vi "Configure Acquisition.vi"(7 "Continuous Storage (T: Enable)":bool=TRUE, 8 "error in (no error)":errorcluster, 10 "Sample Rate (0: 62.5 mHz)":u16(ring) items=["62.5 mHz", "125 mHz", "250 mHz", "500 mHz", "1 Hz", "2 Hz", "4 Hz", "8Hz", "16 Hz", "32 Hz", "64 Hz", "128 Hz", "256 Hz", "512 Hz", "Trigger "], 11 "VISA resource name":refnum<visa-resource-name>) -> (0 "error out":errorcluster, 3 "VISA resource name out":refnum<visa-resource-name>)   [LabVIEW 2020, in "Stanford Research 830.lvlib"]
doc: "Configures the storage of the acquired data in the internal buffer.\n\n<B>Note:</B>\n\nThis VI configures how the data is acquired and stored from the display to the internal buffer of the instrument."
uses:
  Stanford Research 830.lvlib
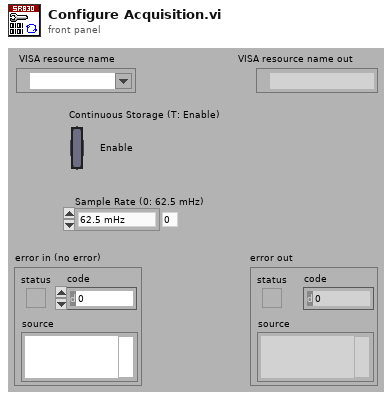
[diagram p1: front panel]
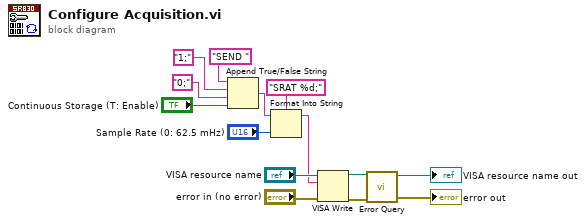
[diagram p0: block diagram]
diagram:
  n1 = Append True/False String(1:"Continuous Storage (T: Enable)", 2:"0;" ("false string"), 3:"1;" ("true string"), 4:"SEND " ("string (\"\")")) -> (0:w7:string)
  n2 = Format Into String(format string="SRAT %d;", initial string=w7, "Sample Rate (0: 62.5 mHz)") -> (resulting string=w5:string)  [unwired: 1 in, 1 out]
  n3 = VISA Write(VISA resource name="VISA resource name", write buffer=w5, error in (no error)="error in (no error)") -> (VISA resource name out=w4:refnum<visa-resource-name>, error out=w3:errorcluster)  [unwired: 1 out]
  n4 = call "Error Query.vi"("error in (no error)"=w3, "VISA resource name"=w4) -> ("error out"=→"error out":errorcluster, "VISA resource name out"=→"VISA resource name out":refnum<visa-resource-name>)  [unwired: 7 in, 1 out]
